vi "ex_4.vi"() -> ()   [LabVIEW 2020]
uses:
  #typedef_hexahedron_parameteres.ctl
panel:
  out "error out":errorcluster
  in  "error in (no error)":errorcluster
  in  "Parameteres of hexahedron  2":T1
  out "Area of hexahedron 2":dbl
  out "Area of hexahedron":dbl format="%#_13g"
  in  "Parameteres of hexahedron":T1
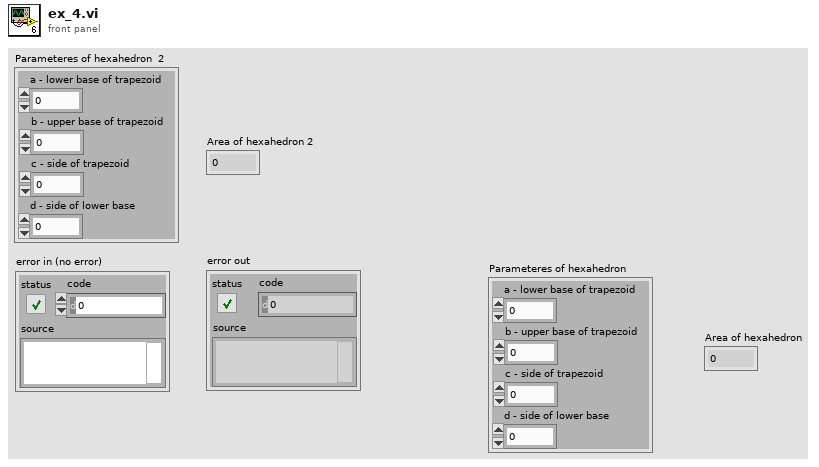
[diagram p1: front panel]
types:
  T1 = typedef "#typedef_hexahedron_parameteres.ctl" = cluster{"a - lower base of trapezoid ":dbl, "b - upper base of trapezoid":dbl, "c - side of trapezoid ":dbl, "d - side of lower base ":dbl}
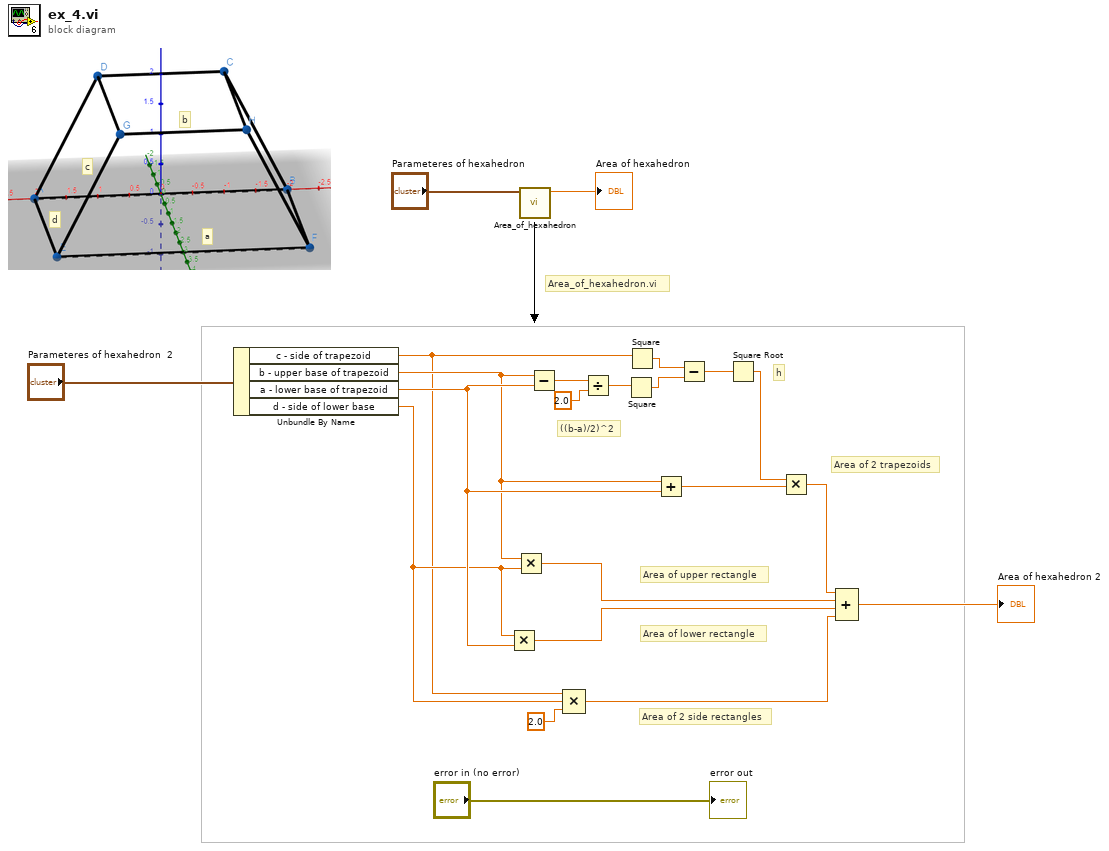
[diagram p0: block diagram]
diagram:
  # "Area_of_hexahedron.vi"
  # "Area of 2 side rectangles"
  # "Area of lower rectangle"
  # "Area of upper rectangle"
  # "Area of 2 trapezoids"
  # "h"
  # "((b-a)/2)^2"
  # "d"
  # "c"
  # "b"
  # "a"
  n1 = Unbundle By Name("Parameteres of hexahedron  2") -> ("c - side of trapezoid"=w11:dbl, "b - upper base of trapezoid"=w13:dbl, "a - lower base of trapezoid"=w15:dbl, "d - side of lower base"=w14:dbl)
  n2 = Multiply(x=w14, y=w15) -> (x*y=w18:dbl)
  n3 = Multiply(x=w13, y=w14) -> (x*y=w17:dbl)
  n4 = call "Area_of_hexahedron.vi"("Parameteres of hexahedron"="Parameteres of hexahedron") -> ("Area of hexahedron"=→"Area of hexahedron":dbl)  [unwired: 9 in, 1 out]
  n5 = Subtract(x=w13, y=w15) -> (x-y=w3:dbl)
  n6 = Compound Arithmetic op=MULTIPLY(w11, w14, 2.0 ("value")) -> (w19:dbl)
  n7 = Divide(x=w3, y=2.0) -> (x/y=w5:dbl)
  n8 = Square(x=w5) -> (x^2=w7:dbl)
  n9 = Square(x=w11) -> (x^2=w6:dbl)
  n10 = Add(x=w13, y=w15) -> (x+y=w9:dbl)
  n11 = Subtract(x=w6, y=w7) -> (x-y=w8:dbl)
  n12 = Square Root(x=w8) -> (sqrt(x)=w10:dbl)
  n13 = Multiply(x=w10, y=w9) -> (x*y=w16:dbl)
  n14 = Compound Arithmetic op=ADD(w16, w17, w18, w19) -> (→"Area of hexahedron 2":dbl)
  "error out" <- "error in (no error)"
